vi "ParseForTestNames.vi"(10 "Instruments":cluster{"Folder Path":path, "tags":string[]}[](array[cluster])) -> (2 "tests":string[](array[string]), 3 "instruments":string[](array[string]))   [LabVIEW 2022 SP3]
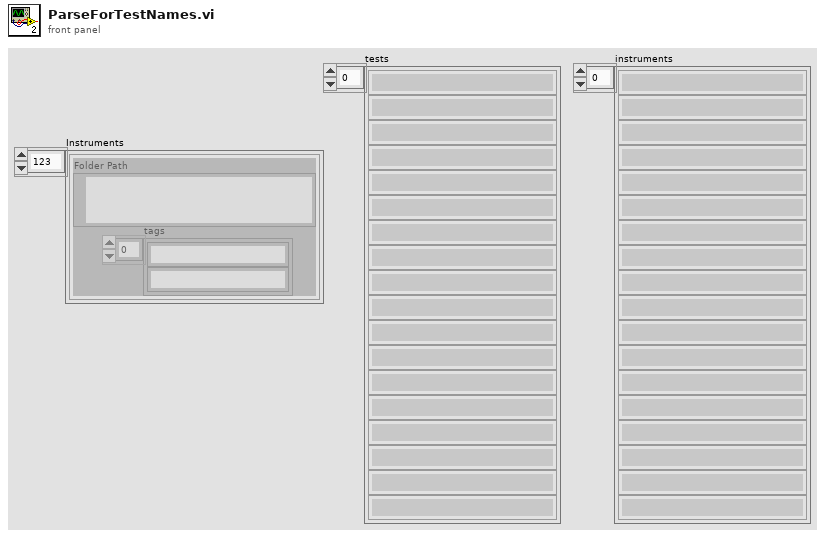
[diagram p1: front panel]
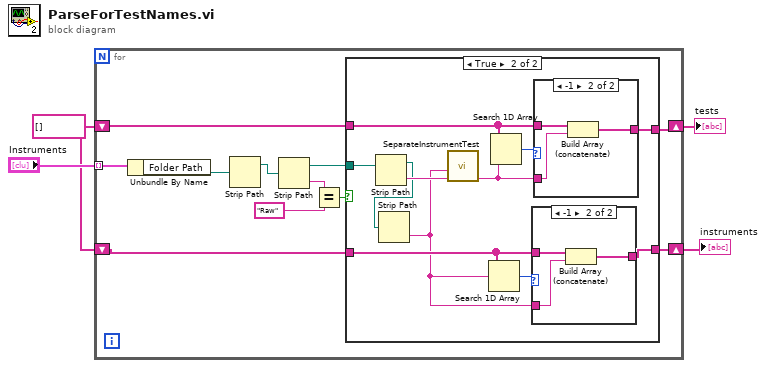
[diagram p0: block diagram]
diagram:
  w2 = string[] []
  n1 = for {
    tunnel: "Instruments" -> [w15] mode=indexing
    shift-right: [w9] -> w3
    shift-left: w2 -> [w8]
    shift-right: [w6] -> w1
    shift-left: w2 -> [w5]
    n2 = Unbundle By Name(w15) -> ("Folder Path"=w14:path)
    n3 = Strip Path(path=w14) -> (stripped path=w13:path)  [unwired: 1 out]
    n4 = Strip Path(path=w13) -> (stripped path=w10:path, name=w12:string)
    n5 = Equal?(x=w12, y="Raw") -> (x = y?=w7:bool)
    n6 = case shown="True" w7 {
      tunnel: w10 -> [_ w28]
      tunnel: [w17 w27] -> w9
      tunnel: w8 -> [w17 w26]
      tunnel: [w16 w21] -> w6
      tunnel: w5 -> [w16 w20]
      frame False {
      }
      frame True {
        n7 = Strip Path(path=w28) -> (stripped path=w23:path, name=w25:string)
        n8 = Strip Path(path=w23) -> (name=w19:string)  [unwired: 1 out]
        n9 = call "SeparateInstrumentTest.vi"("test in"=w25, "Instrument in"=w19) -> ("Instrument -- test out"=w18:string)  [unwired: 5 in, 4 out]
        n10 = Search 1D Array(1D array=w20, element=w19) -> (index of element=w22:i32)  [unwired: 1 in]
        n11 = Search 1D Array(1D array=w26, element=w18) -> (index of element=w24:i32)  [unwired: 1 in]
        n12 = case shown="-1" w22 {
          tunnel: w19 -> [_ w32]
          tunnel: [w29 w31] -> w21
          tunnel: w20 -> [w29 w30]
          frame Default {
          }
          frame -1 {
            n13 = Build Array (concatenate)(w30, w32) -> (w31:string[])
          }
        }
        n14 = case shown="-1" w24 {
          tunnel: [w33 w36] -> w27
          tunnel: w26 -> [w33 w35]
          tunnel: w18 -> [_ w34]
          frame Default {
          }
          frame -1 {
            n15 = Build Array (concatenate)(w35, w34) -> (w36:string[])
          }
        }
      }
    }
  }
  "tests" <- w3
  "instruments" <- w1
